vi "Register for Events (Object).vi"(8 "error in (no error)":errorcluster, 9 "PyObject.lvclass":refnum<class "PyObject.lvclass">, 11 "JKI_Python_Server in":refnum<class "Server.lvclass">) -> (0 "error out":errorcluster, 1 "Python Event":T1, 3 "JKI_Python_Server out":refnum<class "Server.lvclass">)   [LabVIEW 2013, in "JKI_Python_Bridge_for_LV.lvlib" / "Server.lvclass"]
uses:
  Server.lvclass
  Type Definitions/Python Method Call - Event Registration.ctl
  Call/Call.lvclass
  Type Definitions/Public Events - Cluster.ctl
  PyObject/PyObject.lvclass
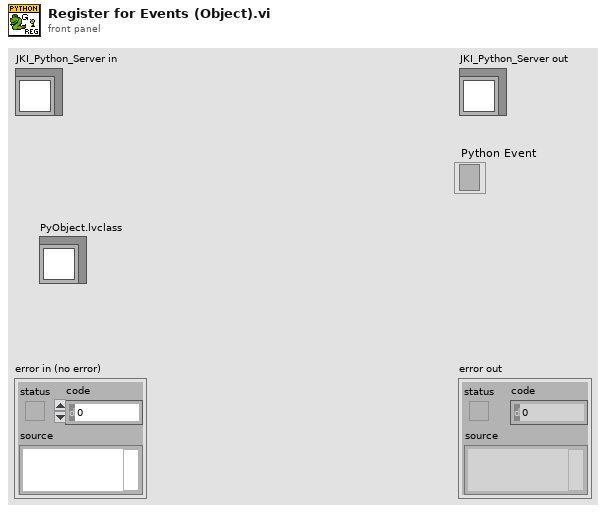
[diagram p1: front panel]
types:
  T1 = typedef "JKI_Python_Bridge_for_LV.lvlib/Server.lvclass/Python Method Call - Event Registration.ctl" = refnum<event-registration>
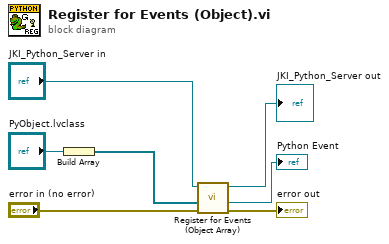
[diagram p0: block diagram]
diagram:
  n1 = Build Array("PyObject.lvclass") -> (w6:refnum<class "PyObject.lvclass">[])
  n2 = call "Register for Events (Object Array).vi"("error in (no error)"="error in (no error)", "PyObject []"=w6, "JKI_Python_Server in"="JKI_Python_Server in") -> ("error out"=→"error out":errorcluster, "Python Event"=→"Python Event":T1, "JKI_Python_Server out"=→"JKI_Python_Server out":refnum<class "Server.lvclass">)  [unwired: 6 in]
